vi "MindwaveClose.vi"(1 "error in (no error)":errorcluster, 2 "VISA resource name input":refnum<visa-resource-name>) -> ()   [LabVIEW 2011, in "Neurosky.lvlib"]
uses:
  Users/Isaias/Documents/GitHub/Neurosky/Neurosky.lvlib
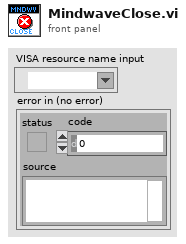
[diagram p1: front panel]
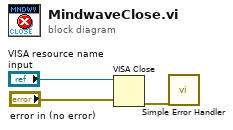
[diagram p0: block diagram]
diagram:
  n1 = VISA Close(VISA resource name="VISA resource name input", error in (no error)="error in (no error)") -> (error out=w1:errorcluster)
  n2 = call <vilib>:"Simple Error Handler.vi"("error in (no error)"=w1) -> ()  [unwired: 4 in, 5 out]
